vi "Set Type Thermocouple.vi"(6 "Compensation":u16(ring) items=["Compensated", "No Compensated"], 7 "Temperature Unit":u16(ring) items=["Celsius", "Fahrenheit", "Kelvin"], 8 "error in (no error)":errorcluster, 9 "Thermocouple type":u16(ring) items=["J", "K", "T", "S", "B", "E", "N", "C", "L"], 10 "Channel":u16(ring) items=["A1"=0, "A2"=1, "A3"=2, "A4"=3, "A5"=4, "A6"=5, "A7"=6, "A8"=7, "A9"=8, "A10"=9, "K1"=200, "K2"=201, "K3"=202, "K4"=203, "FA1"=204, "FA2"=205, "FA3"=206, "FA4"=207], 11 "VISA resource name":refnum<visa-resource-name>) -> (0 "error out":errorcluster, 3 "VISA resource name out":refnum<visa-resource-name>)   [LabVIEW 2017, in "Sefram DAS220.lvlib"]
doc: "Set input type as thermocouple."
uses:
  <instrlib>/Sefram DAS220/Sefram DAS220.lvlib
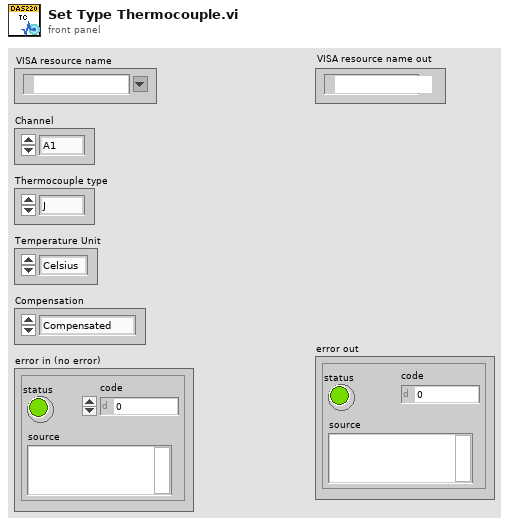
[diagram p1: front panel]
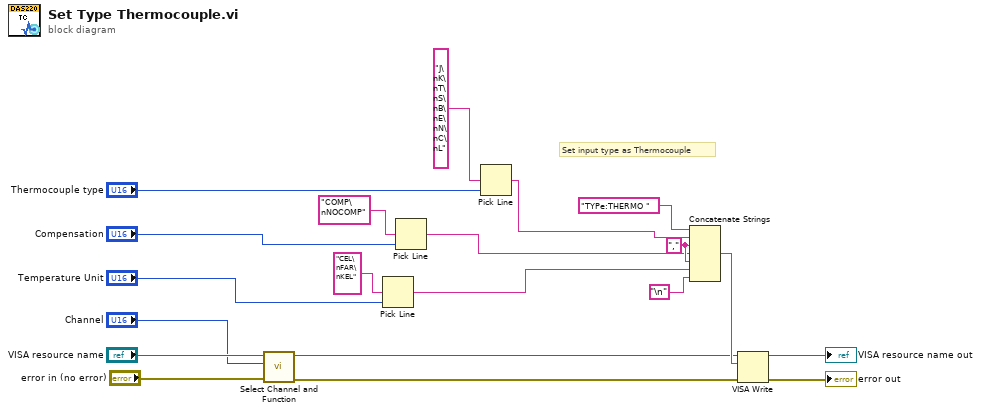
[diagram p0: block diagram]
diagram:
  w16 = "," ("string")
  # "Set input type as Thermocouple"
  n1 = call <instrlib>:"Select Channel and Function.vi"("error in (no error)"="error in (no error)", "Channel"="Channel", "VISA resource name"="VISA resource name") -> ("error out"=w2:errorcluster, "VISA resource name out"=w13:refnum<visa-resource-name>)  [unwired: 7 in]
  n2 = Pick Line(multi-line string="CEL\nFAR\nKEL", line index="Temperature Unit") -> (output string=w6:string)  [unwired: 1 in]
  n3 = Pick Line(multi-line string="COMP\nNOCOMP", line index="Compensation") -> (output string=w3:string)  [unwired: 1 in]
  n4 = Pick Line(multi-line string="J\nK\nT\nS\nB\nE\nN\nC\nL", line index="Thermocouple type") -> (output string=w9:string)  [unwired: 1 in]
  n5 = Concatenate Strings("TYPe:THERMO " ("string"), w9, w16, w3, w16, w6, "\n") -> (w20:string)
  n6 = VISA Write(VISA resource name=w13, write buffer=w20, error in (no error)=w2) -> (VISA resource name out=→"VISA resource name out":refnum<visa-resource-name>, error out=→"error out":errorcluster)  [unwired: 1 out]
